vi "Get Data Variant.vi"(8 "error in (no error)":errorcluster, 11 "UDP Rx Transfer Configuration in":refnum<class "UDP Transfer Rx Configuration.lvclass">) -> (0 "error out":errorcluster, 1 "data version":T1, 2 "data":variant, 3 "UDP Rx Transfer Configuration out":refnum<class "UDP Transfer Rx Configuration.lvclass">)   [LabVIEW 2023, in "UDP.lvlib" / "UDP Transfer Rx Configuration.lvclass"]
uses:
  UDP Transfer Rx Configuration.lvclass
  Users/Public/Documents/National Instruments/NI VeriStand 2023/Custom Devices/Data Sharing Framework/Linux_x64/DSF Core.lvlibp/Typedefs/DSF Version Info.ctl
  UDP Transfer Rx Configuration.lvclass/UDP Transfer Rx Configuration.ctl
  Users/Public/Documents/National Instruments/NI VeriStand 2023/Custom Devices/Data Sharing Framework/Linux_x64/DSF Core.lvlibp
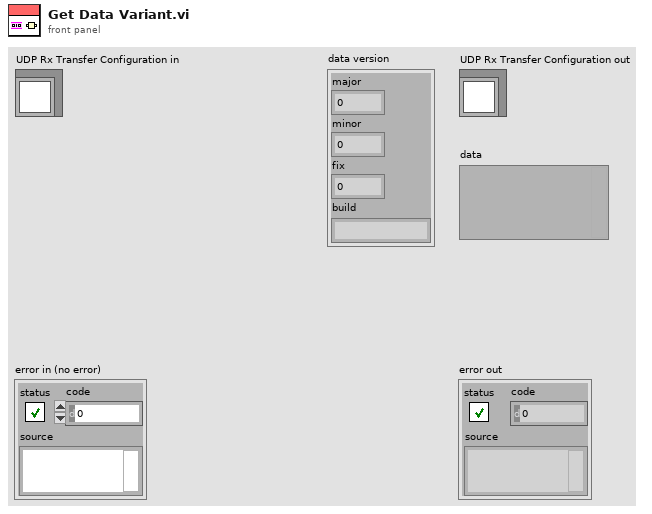
[diagram p1: front panel]
types:
  T1 = typedef "DSF Core.lvlibp/DSF Version Info.ctl" = cluster{"major":u32, "minor":u32, "fix":u32, "build":string}
  T2 = typedef "UDP.lvlib/UDP Transfer Rx Configuration.lvclass/Rx Transfer Settings.ctl" = cluster{"address":u32, "port":u16}
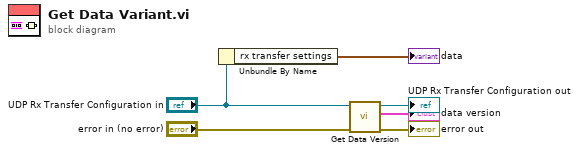
[diagram p0: block diagram]
diagram:
  n1 = Unbundle By Name("UDP Rx Transfer Configuration in") -> ("rx transfer settings"=→"data":T2)
  n2 = call-dynamic "Get Data Version.vi"("error in (no error)"="error in (no error)", "UDP Rx Transfer Configuration in"="UDP Rx Transfer Configuration in") -> ("error out"=→"error out":errorcluster, "data version"=→"data version":T1, "UDP Rx Transfer Configuration out"=→"UDP Rx Transfer Configuration out":refnum<class "UDP Transfer Rx Configuration.lvclass">)  [unwired: 7 in]
